vi "flash_cycle(SubVI).vi"(6 "Boolean in":bool, 9 "Number of cyles\nbetween flashes":i32, 10 "Numeric":i32, 11 "Flash lamp?":bool) -> (3 "Boolean out":bool)   [LabVIEW 2012]
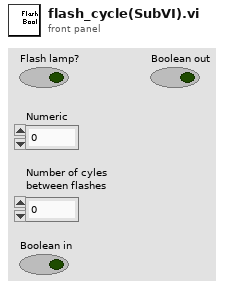
[diagram p1: front panel]
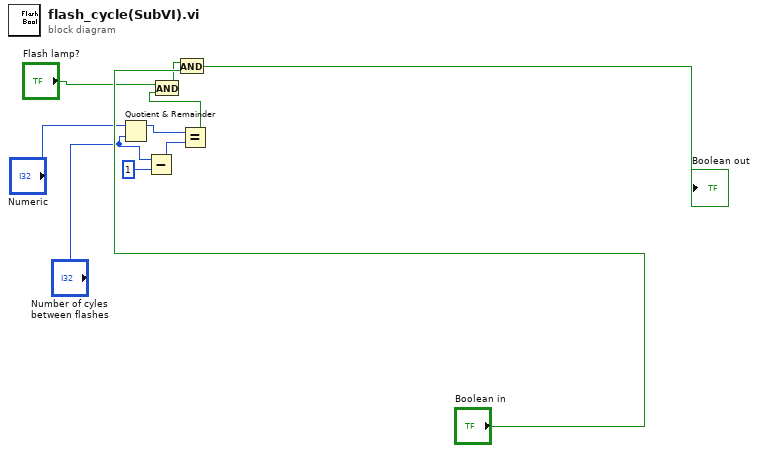
[diagram p0: block diagram]
diagram:
  n1 = Quotient & Remainder(x="Numeric", y="Number of cyles\nbetween flashes") -> (x-y*floor(x/y)=w1:i32)  [unwired: 1 out]
  n2 = Subtract(x="Number of cyles\nbetween flashes", y=1) -> (x-y=w4:i32)
  n3 = Equal?(x=w1, y=w4) -> (x = y?=w5:bool)
  n4 = And(x="Flash lamp?", y=w5) -> (x .and. y?=w8:bool)
  n5 = And(x=w8, y="Boolean in") -> (x .and. y?=→"Boolean out":bool)
